vi "current viewer - multiple.vi"() -> ()   [LabVIEW 2018]
panel:
  in  "desired motion":i32
  out "Motor Current Versus Time":sgl[][](graph)
  # "v1.01"
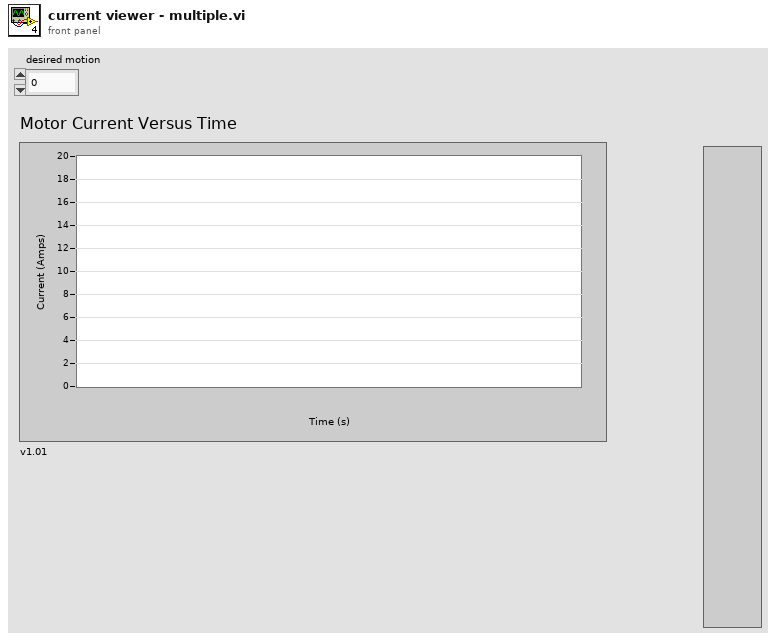
[diagram p1: front panel]
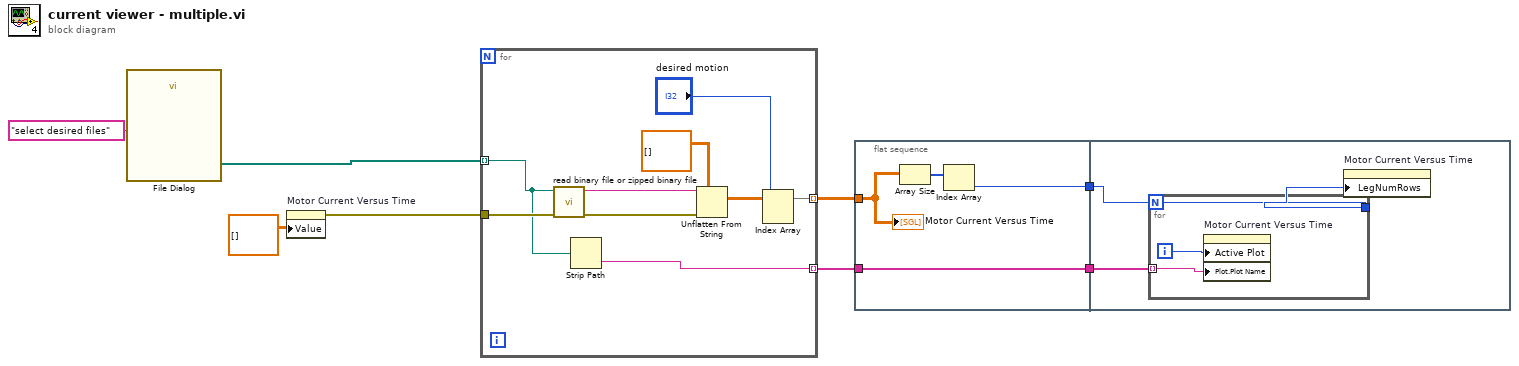
[diagram p0: block diagram]
diagram:
  n1 = call "File Dialog"("prompt"="select desired files") -> ("selected paths"=w3:path[])  [unwired: 11 in, 3 out]
  n2 = property on="Motor Current Versus Time" class="WFGraph (严格)"("Value"=sgl[][] [] ("Motor Current Versus Time")) -> (error out=w6:errorcluster)  [unwired: 2 in, 1 out]
  n3 = for {
    tunnel: w6 -> [w17]
    tunnel: [w13] -> w5 mode=indexing
    tunnel: w3 -> [w10] mode=indexing
    tunnel: [w9] -> w1 mode=indexing
    n4 = call "read binary file or zipped binary file.vi"("error in"=w17, "File"=w10) -> ("error out"=w15:errorcluster, "data"=w11:string)  [unwired: 8 in]
    n5 = Strip Path(path=w10) -> (name=w9:string)  [unwired: 1 out]
    n6 = Unflatten From String(type=sgl[][] [], binary string=w11, error in (no error)=w15) -> (value=w14:sgl[][])  [unwired: 2 in, 2 out]
    n7 = Index Array(array=w14, index (row)="desired motion") -> (element=w13:sgl[])  [unwired: 1 in]
  }
  n8 = flat-sequence {
    tunnel: w5 -> [w20]
    tunnel: [w19] -> w7
    tunnel: [w18] -> w2
    tunnel: w1 -> [w18]
    tunnel: w7 -> [w24]
    tunnel: w2 -> [w22]
    frame #0 {
      n9 = Array Size(array=w20) -> (size(s)=w21:i32[])
      n10 = Index Array(array=w21) -> (element=w19:i32)  [unwired: 1 in]
      "Motor Current Versus Time" <- w20
    }
    frame #1 {
      n11 = for {
        N: w24 -> [w27]
        tunnel: [w27] -> w23
        tunnel: w22 -> [w25] mode=indexing
        i -> [w26]
        n12 = property on="Motor Current Versus Time" class="WFGraph (严格)"("Active Plot"=w26, "Plot.Plot Name"=w25) -> ()  [unwired: 2 in, 2 out]
      }
      n13 = property on="Motor Current Versus Time" class="WFGraph (严格)"("LegNumRows"=w23) -> ()  [unwired: 2 in, 2 out]
    }
  }
